vi "Process File.vi"(8 "error in (no error)":errorcluster, 10 "File":refnum<class "Acquired Result.lvclass">, 11 "NHMFL Synthesizer in":refnum<class "NHMFL Synthesizer.lvclass">) -> (0 "error out":errorcluster, 2 "File out":refnum<class "Acquired Result.lvclass">, 3 "NHMFL Synthesizer out":refnum<class "NHMFL Synthesizer.lvclass">)   [LabVIEW 2016, in "NHMFL Synthesizer.lvclass"]
uses:
  NHMFL Synthesizer.lvclass
  NHMFL_Core/Libraries/Instruments/Results/Acquired Result/Acquired Result.lvclass
  NHMFL Synthesizer.lvclass/NHMFL Synthesizer.ctl
  Read NHMFL Synthesizer Configuration.vi
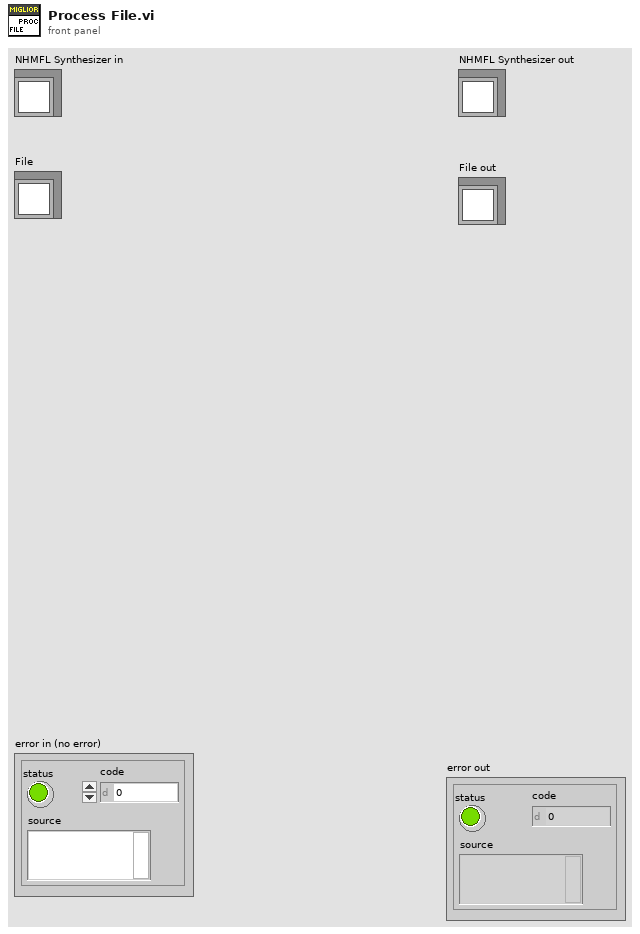
[diagram p1: front panel]
types:
  T1 = enum16{"open", "open or create", "create or replace", "create", "open (read-only)"}
  T2 = typedef "NHMFL Synthesizer Configuration.ctl" = cluster{"DAQmx Device":tag, "Variable amplitude frequency":dbl, "Fixed amplitude frequency":dbl, "Amplitude":dbl, "Clock multiplier":i32, "Channel names (variable F)":string[], "Channel names (fixed F)":string[], "Group":string, "Auto-update other modules":bool, "Recorder module":string, "Lock-in module ":string}
  T3 = typedef "Lockin Parameters.ctl" = cluster{"Frequency":dbl, "Phase":dbl, "Syncronous":bool, "Points per sine wave":i32, "DDS":bool, "Frequency word":u32, "Phase word":u32, "DDS modulus":i64, "DDS clock":dbl}
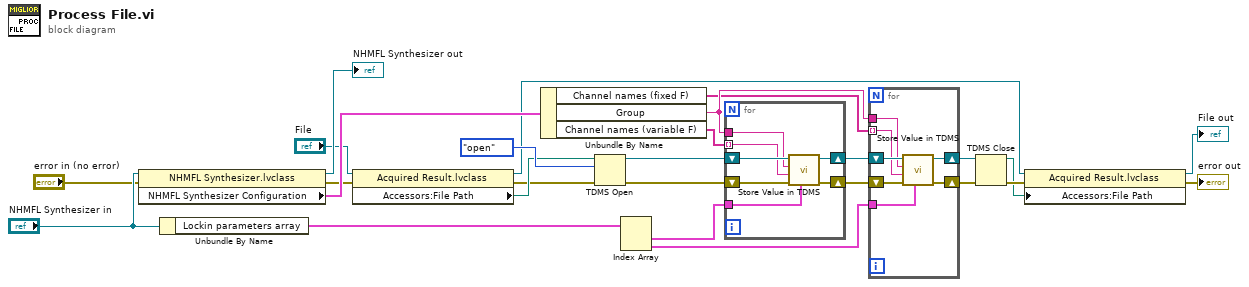
[diagram p0: block diagram]
diagram:
  n1 = property class="NHMFL Synthesizer.lvclass"(reference="NHMFL Synthesizer in", error in="error in (no error)") -> (reference out=→"NHMFL Synthesizer out":refnum<class "NHMFL Synthesizer.lvclass">, error out=w7:errorcluster, "NHMFL Synthesizer Configuration"=w22:T2)
  n2 = Unbundle By Name("NHMFL Synthesizer in") -> ("Lockin parameters array"=w18:T3[])
  n3 = property class="Acquired Result.lvclass"(reference="File", error in=w7) -> (reference out=w1:refnum<class "Acquired Result.lvclass">, error out=w6:errorcluster, "Accessors:File Path"=w8:path)
  n4 = Unbundle By Name(w22) -> ("Channel names (fixed F)"=w10:string[], "Group"=w15:string, "Channel names (variable F)"=w21:string[])
  n5 = TDMS Open(8:w6, 10:T1."open" ("operation (0:open)"), 11:w8) -> (0:w19:errorcluster, 3:w20:refnum<k34>)  [unwired: 4 in]
  n6 = Index Array(array=w18) -> (element #1=w17:T3, element #2=w16:T3)  [unwired: 2 in]
  n7 = for {
    tunnel: w21 -> [w29] mode=indexing
    shift-right: [w32] -> w13
    shift-left: w20 -> [w33]
    shift-right: [w31] -> w14
    shift-left: w19 -> [w28]
    tunnel: w15 -> [w30]
    tunnel: w17 -> [w27]
    n8 = call "Store Value in TDMS.vi"("Value"=w27, "Error In"=w28, "channel name"=w29, "group name"=w30, "tdms file"=w33) -> ("Error Out"=w31:errorcluster, "tdms file out"=w32:refnum<k34>)  [unwired: 3 in, 2 out]
  }
  n9 = for {
    tunnel: w10 -> [w36] mode=indexing
    shift-right: [w39] -> w12
    shift-left: w13 -> [w40]
    shift-right: [w38] -> w11
    shift-left: w14 -> [w35]
    tunnel: w15 -> [w37]
    tunnel: w16 -> [w34]
    n10 = call "Store Value in TDMS.vi"("Value"=w34, "Error In"=w35, "channel name"=w36, "group name"=w37, "tdms file"=w40) -> ("Error Out"=w38:errorcluster, "tdms file out"=w39:refnum<k34>)  [unwired: 3 in, 2 out]
  }
  n11 = TDMS Close(8:w11, 11:w12) -> (0:w5:errorcluster, 3:w2:path)
  n12 = property class="Acquired Result.lvclass"(reference=w1, error in=w5, "Accessors:File Path"=w2) -> (reference out=→"File out":refnum<class "Acquired Result.lvclass">, error out=→"error out":errorcluster)
